vi "StringToHex.vi"(11 "字符串":string) -> (3 "数组":u16[](array[numeric]) format="%04xH")   [LabVIEW 2016, in "氨氮.lvlib"]
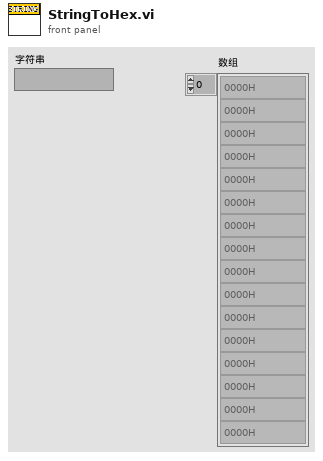
[diagram p1: front panel]
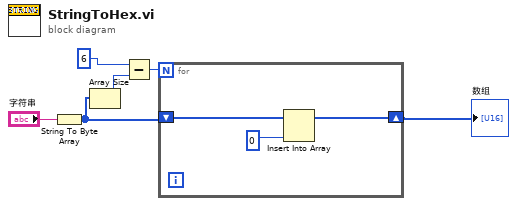
[diagram p0: block diagram]
diagram:
  n1 = String To Byte Array(string="字符串") -> (unsigned byte array=w4:u8[])
  n2 = Array Size(array=w4) -> (size(s)=w3:i32)
  n3 = Subtract(x=6, y=w3) -> (x-y=w1:i32)
  n4 = for {
    N: w1 -> [_]
    shift-right: [w8] -> w5
    shift-left: w4 -> [w7]
    n5 = Insert Into Array(array=w7, new element=u8 0 ("新元素/子数组")) -> (w8:u8[])  [unwired: 1 in]
  }
  "数组" <- w5
